vi "VI Tree.vi"   [LabVIEW 2021, in "Keithley 2182.lvlib"]
doc: "This is the instrument driver for the Keithley 2182. The VI Tree displays all the user-callable VIs of the instrument driver in an organized table."
uses:
  <instrlib>/Keithley 2182/Keithley 2182.lvlib
panel:
  # "(c) 2017-2018 National Instruments.  ALL RIGHTS RESERVED."
  # "SEE DIAGRAM\nFOR VI TREE."
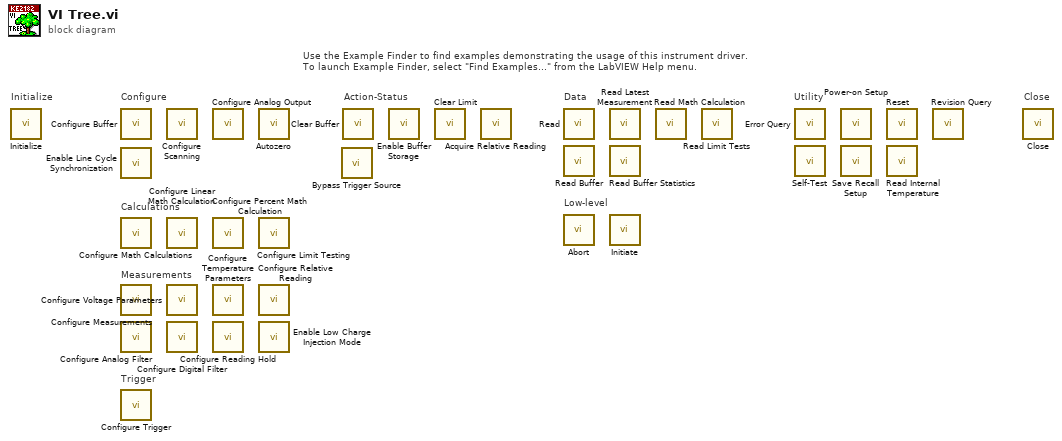
[diagram p0: block diagram]
diagram:
  # "Close"
  # "Utility"
  # "Low-level"
  # "Data"
  # "Trigger"
  # "Measurements"
  # "Calculations"
  # "Configure"
  # "Action-Status"
  # "Initialize"
  # "Use the Example Finder to find examples demonstrating the usage of this instrument driver.\nTo launch Example Finder, select \"Find Examples...\" from the LabVIEW Help menu."
  n1 = call <instrlib>:"Initialize.vi"() -> ()  [unwired: 10 in, 2 out]
  n2 = call <instrlib>:"Configure Buffer.vi"() -> ()  [unwired: 10 in, 2 out]
  n3 = call <instrlib>:"Enable Line Cycle Synchronization.vi"() -> ()  [unwired: 10 in, 2 out]
  n4 = call <instrlib>:"Configure Math Calculations.vi"() -> ()  [unwired: 10 in, 2 out]
  n5 = call <instrlib>:"Configure Measurements.vi"() -> ()  [unwired: 14 in, 2 out]
  n6 = call <instrlib>:"Configure Analog Filter.vi"() -> ()  [unwired: 14 in, 2 out]
  n7 = call <instrlib>:"Configure Trigger.vi"() -> ()  [unwired: 14 in, 2 out]
  n8 = call <instrlib>:"Configure Scanning.vi"() -> ()  [unwired: 10 in, 2 out]
  n9 = call <instrlib>:"Configure Linear Math Calculation.vi"() -> ()  [unwired: 10 in, 2 out]
  n10 = call <instrlib>:"Configure Voltage Parameters.vi"() -> ()  [unwired: 14 in, 2 out]
  n11 = call <instrlib>:"Configure Digital Filter.vi"() -> ()  [unwired: 14 in, 2 out]
  n12 = call <instrlib>:"Configure Analog Output.vi"() -> ()  [unwired: 10 in, 2 out]
  n13 = call <instrlib>:"Configure Percent Math Calculation.vi"() -> ()  [unwired: 10 in, 2 out]
  n14 = call <instrlib>:"Configure Temperature Parameters.vi"() -> ()  [unwired: 14 in, 2 out]
  n15 = call <instrlib>:"Configure Reading Hold.vi"() -> ()  [unwired: 10 in, 2 out]
  n16 = call <instrlib>:"Autozero.vi"() -> ()  [unwired: 10 in, 2 out]
  n17 = call <instrlib>:"Configure Limit Testing.vi"() -> ()  [unwired: 14 in, 2 out]
  n18 = call <instrlib>:"Configure Relative Reading.vi"() -> ()  [unwired: 14 in, 2 out]
  n19 = call <instrlib>:"Enable Low Charge Injection Mode.vi"() -> ()  [unwired: 10 in, 2 out]
  n20 = call <instrlib>:"Bypass Trigger Source.vi"() -> ()  [unwired: 10 in, 2 out]
  n21 = call <instrlib>:"Clear Buffer.vi"() -> ()  [unwired: 10 in, 2 out]
  n22 = call <instrlib>:"Enable Buffer Storage.vi"() -> ()  [unwired: 10 in, 2 out]
  n23 = call <instrlib>:"Clear Limit.vi"() -> ()  [unwired: 10 in, 2 out]
  n24 = call <instrlib>:"Acquire Relative Reading.vi"() -> ()  [unwired: 14 in, 2 out]
  n25 = call <instrlib>:"Read.vi"() -> ()  [unwired: 8 in, 4 out]
  n26 = call <instrlib>:"Read Buffer.vi"() -> ()  [unwired: 8 in, 4 out]
  n27 = call <instrlib>:"Abort.vi"() -> ()  [unwired: 10 in, 2 out]
  n28 = call <instrlib>:"Read Latest Measurement.vi"() -> ()  [unwired: 8 in, 4 out]
  n29 = call <instrlib>:"Read Buffer Statistics.vi"() -> ()  [unwired: 6 in, 6 out]
  n30 = call <instrlib>:"Initiate.vi"() -> ()  [unwired: 10 in, 2 out]
  n31 = call <instrlib>:"Read Math Calculation.vi"() -> ()  [unwired: 8 in, 4 out]
  n32 = call <instrlib>:"Read Limit Tests.vi"() -> ()  [unwired: 12 in, 4 out]
  n33 = call <instrlib>:"Error Query.vi"() -> ()  [unwired: 8 in, 4 out]
  n34 = call <instrlib>:"Self-Test.vi"() -> ()  [unwired: 8 in, 4 out]
  n35 = call <instrlib>:"Power-on Setup.vi"() -> ()  [unwired: 10 in, 2 out]
  n36 = call <instrlib>:"Save Recall Setup.vi"() -> ()  [unwired: 10 in, 2 out]
  n37 = call <instrlib>:"Reset.vi"() -> ()  [unwired: 10 in, 2 out]
  n38 = call <instrlib>:"Read Internal Temperature.vi"() -> ()  [unwired: 9 in, 3 out]
  n39 = call <instrlib>:"Revision Query.vi"() -> ()  [unwired: 8 in, 4 out]
  n40 = call <instrlib>:"Close.vi"() -> ()  [unwired: 11 in, 1 out]
